vi "Initialize MeasurementLink Session.vi"(7 "remote connection options":T2, 8 "error in":errorcluster, 9 "initialize and close session behavior":T1, 10 "session initialization parameters":T3, 11 "session factory in":refnum<class "KeysightDmm.lvclass">) -> (0 "error out":errorcluster, 2 "session out":variant, 3 "session factory out":refnum<class "KeysightDmm.lvclass">)   [LabVIEW 2021, in "KeysightDmm.lvclass"]
doc: "Creates a new session using the provided <b>session initialization parameters</b>. If the session represents a remote session, <b>initialize and close session behavior</b> determines whether creating the local session creates a new session on the server or attaches to an existing session on the server."
uses:
  KeysightDmm.lvclass
  <vilib>/Plug-In SDKs/Sessions/Instrument/ISession Factory/Session Initialization Parameters.ctl
  <vilib>/Plug-In SDKs/Sessions/Instrument/ISession Factory/Remote Connection Options.ctl
  <vilib>/Plug-In SDKs/Sessions/Instrument/ISession Factory/Initialize and Close Session Behavior.ctl
  KeysightDmm.lvclass/KeysightDmm.ctl
  <vilib>/Plug-In SDKs/Sessions/Instrument/ISession Factory/ISession Factory.lvclass
  <instrlib>/Agilent 34401/Public/Initialize.vi
  <instrlib>/Agilent 34401/Agilent 34401.lvlib
  SubVI/Get VISA gRPC Open Close Behavior.vi
  <vilib>/NI-VISA/VISA Open for gRPC Session.vi
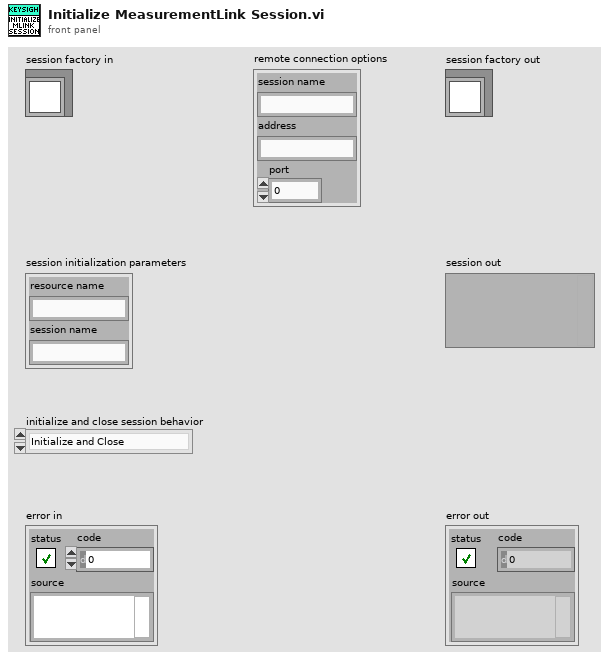
[diagram p1: front panel]
types:
  T1 = typedef "NI Session Management Instrument.lvlib/ISession Factory.lvclass/Initialize and Close Session Behavior.ctl" = enum16{"Initialize and Close", "Attach and Detach", "Initialize and Detach", "Attach and Close"}
  T2 = typedef "NI Session Management Instrument.lvlib/ISession Factory.lvclass/Remote Connection Options.ctl" = cluster{"session name":string, "address":string, "port":u32}
  T3 = typedef "NI Session Management Instrument.lvlib/ISession Factory.lvclass/Session Initialization Parameters.ctl" = cluster{"resource name":string, "session name":string}
  T4 = typedef "VISA gRPC Open Close Behavior.ctl" = enum16{"Auto", "Initialize and Close", "Attach and Detach", "Initialize and Detach", "Attach and Close"}
  T5 = cluster{"Baud Rate":u32, "Parity":u16, "Data Bits":u16}
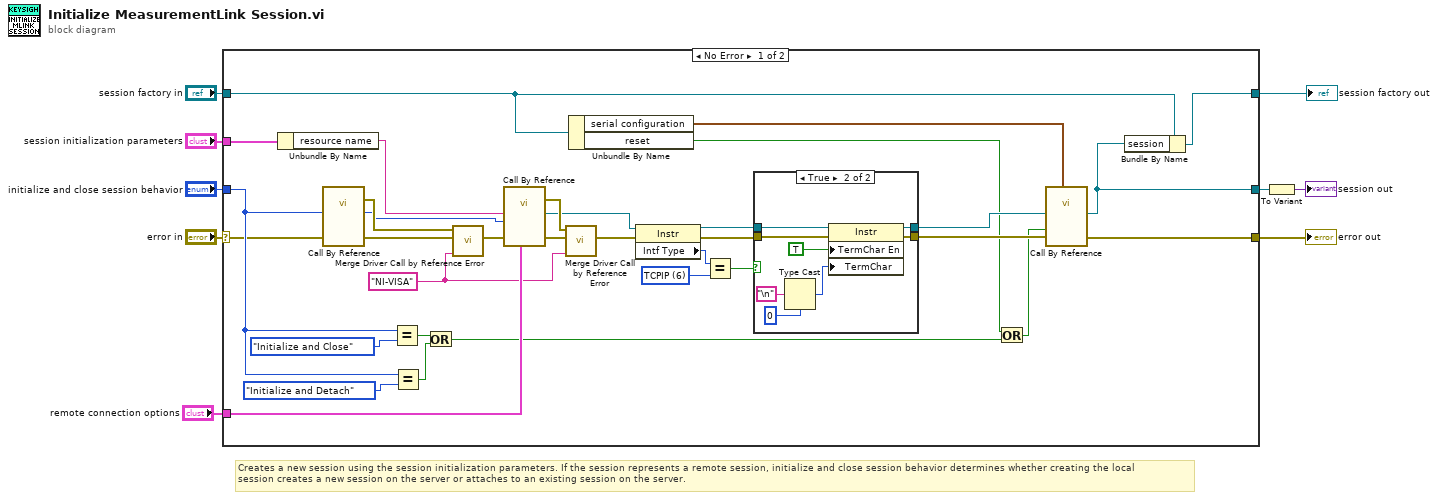
[diagram p0: block diagram]
diagram:
  # "Creates a new session using the session initialization parameters. If the session represents a remote session, initialize and close session behavior determines whether creating the local \nsession creates a new session on the server or attaches to an existing session on the server."
  n1 = case shown="No Error" "error in" {
    selector: "error in" -> [w37 w53]
    tunnel: [w13 w53] -> w9
    tunnel: "session factory in" -> [w10 w54]
    tunnel: "initialize and close session behavior" -> [w38 _]
    tunnel: "remote connection options" -> [w33 _]
    tunnel: [w11 w54] -> w4
    tunnel: [w12 _] -> w3
    tunnel: "session initialization parameters" -> [w32 _]
    frame No Error {
      w25 = u16 6 items=["GPIB"=1, "VXI"=2, "GPIB-VXI"=3, "Serial"=4, "PXI"=5, "TCPIP"=6, "USB"=7, "FireWire"=9] ("Interface Information:Interface Type")
      w28 = "NI-VISA" ("driver name")
      n2 = Unbundle By Name(w32) -> ("resource name"=w31:string)
      n3 = call-by-ref "?"("initialize session behavior"=w38, "error in (no error)"=w37) -> (error out=w35:errorcluster, "open/close behavior"=w18:T4, 15:"error out"=w36:errorcluster)  [unwired: 14 in, 1 out]
      n4 = Equal?(x=w38, y=Initialize_and_Close_Session_Behavior."Initialize and Close" ("initialize session behavior")) -> (x = y?=w40:bool)
      n5 = Equal?(x=w38, y=Initialize_and_Close_Session_Behavior."Initialize and Detach" ("initialize session behavior")) -> (x = y?=w39:bool)
      n6 = Or(x=w40, y=w39) -> (x .or. y?=w16:bool)
      n7 = call <vilib>:"Merge Driver Call by Reference Error.vi"("driver name"=w28, "called vi error"=w36, "call by ref error"=w35) -> ("error out"=w34:errorcluster)  [unwired: 8 in]
      n8 = call-by-ref "?"("gRPC Options"=w33, "error in (no error)"=w34, "Open/Close Behavior"=w18, "VISA resource name"=w31) -> (error out=w29:errorcluster, 0:"error out"=w30:errorcluster, "VISA resource name out"=w20:refnum<visa-resource-name>)  [unwired: 8 in, 1 out]
      n9 = call <vilib>:"Merge Driver Call by Reference Error.vi"("driver name"=w28, "called vi error"=w30, "call by ref error"=w29) -> ("error out"=w23:errorcluster)  [unwired: 8 in]
      n10 = Unbundle By Name(w10) -> ("serial configuration"=w17:T5, "reset"=w14:bool)
      n11 = property class="Instr"(reference=w20, error in=w23) -> (reference out=w21:refnum<visa-resource-name>, error out=w22:errorcluster, "Intf Type"=w24:u16)
      n12 = Equal?(x=w24, y=w25) -> (x = y?=w19:bool)
      n13 = case shown="True" w19 {
        tunnel: w22 -> [w44 w52]
        tunnel: [w44 w51] -> w27
        tunnel: w21 -> [w43 w50]
        tunnel: [w43 w49] -> w26
        frame False {
        }
        frame True {
          n14 = Type Cast(type=u8 0, x="\n" ("Line Feed Constant")) -> (*(type *) &x=w45:u8)
          n15 = property class="Instr"(reference=w50, error in=w52, "TermChar En"=TRUE ("Message Based Settings:Termination Character Enable"), "TermChar"=w45) -> (reference out=w49:refnum<visa-resource-name>, error out=w51:errorcluster)
        }
      }
      n16 = Or(x=w14, y=w16) -> (x .or. y?=w15:bool)
      n17 = call-by-ref "?"("Serial Configuration"=w17, "error in (no error)"=w27, "Reset (True)"=w15, "VISA resource name"=w26) -> ("error out"=w13:errorcluster, "VISA resource name out"=w12:refnum<visa-resource-name>)  [unwired: 8 in, 2 out]
      n18 = Bundle By Name(cluster=w10, "session"=w12) -> (w11:refnum<class "KeysightDmm.lvclass">)
    }
    frame Error {
    }
  }
  "error out" <- w9
  "session factory out" <- w4
  n19 = To Variant(anything=w3) -> (Variant=→"session out":variant)
